vi "VI Tree.vi"   [LabVIEW 2012, in "Phidget Gyroscope.lvlib"]
doc: "${Gyroscope:VITreeHeader}"
uses:
  <instrlib>/Phidgets/Phidget Gyroscope/Phidget Gyroscope.lvlib
  <instrlib>/Phidgets/Phidget Gyroscope/Public/GyroscopeStart.vi
  <instrlib>/Phidgets/Phidget Gyroscope/Public/GyroscopeOpen.vi
  <instrlib>/Phidgets/Phidget Gyroscope/Public/GyroscopeClose.vi
panel:
  # "(c) 2015 Phidgets Inc..  ALL RIGHTS RESERVED."
  # "SEE DIAGRAM\nFOR VI TREE."
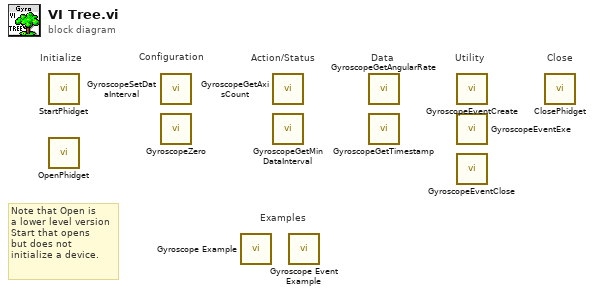
[diagram p0: block diagram]
diagram:
  # "Note that Open is\na lower level version\nStart that opens\nbut does not \ninitialize a device."
  # "Examples"
  # "Configuration"
  # "Utility"
  # "Data"
  # "Action/Status"
  # "Close"
  # "Initialize"
  n1 = call-poly <instrlib>:"StartPhidget.vi"() -> ()  [unwired: 12 in, 4 out]
  n2 = call-poly <instrlib>:"OpenPhidget.vi"() -> ()  [unwired: 8 in, 4 out]
  n3 = call <instrlib>:"GyroscopeSetDataInterval.vi"() -> ()  [unwired: 9 in, 2 out]
  n4 = call <instrlib>:"GyroscopeZero.vi"() -> ()  [unwired: 9 in, 2 out]
  n5 = call <instrlib>:"Gyroscope Example.vi"() -> ()  [unwired: 12 in]
  n6 = call <instrlib>:"GyroscopeGetAxisCount.vi"() -> ()  [unwired: 8 in, 3 out]
  n7 = call <instrlib>:"GyroscopeGetMinDataInterval.vi"() -> ()  [unwired: 8 in, 3 out]
  n8 = call <instrlib>:"Gyroscope Event Example.vi"() -> ()  [unwired: 12 in]
  n9 = call <instrlib>:"GyroscopeGetAngularRate.vi"() -> ()  [unwired: 8 in, 3 out]
  n10 = call <instrlib>:"GyroscopeGetTimestamp.vi"() -> ()  [unwired: 8 in, 3 out]
  n11 = call <instrlib>:"GyroscopeEventCreate.vi"() -> ()  [unwired: 9 in, 3 out]
  n12 = call <instrlib>:"GyroscopeEventExe.vi"() -> ()  [unwired: 8 in, 8 out]
  n13 = call <instrlib>:"GyroscopeEventClose.vi"() -> ()  [unwired: 10 in, 2 out]
  n14 = call-poly <instrlib>:"ClosePhidget.vi"() -> ()  [unwired: 11 in, 1 out]
